vi "Test Helper Loop Restart.vi"(8 "error in (no error)":errorcluster, 11 "Helper Loop Test In":refnum<class "Helper Loop Test.lvclass">) -> (0 "error out":errorcluster, 3 "Helper Loop Test Out":refnum<class "Helper Loop Test.lvclass">)   [LabVIEW 2020, in "Helper Loop Test.lvclass"]
uses:
  Helper Loop Test.lvclass
  C:/Program Files (x86)/National Instruments/LabVIEW 2020/vi.lib/Asteme/LUnit/Test Case.lvclass
  Mock Process/Mock Process.lvclass
  C:/Users/anton/Documents/GitHub/Triarc-Framework/source/Framework/Process/Process.lvclass
  <vilib>/Asteme/LUnit/Test Case.lvclass/Test Case.ctl
  <vilib>/Asteme/LUnit/LUnit Assertion Result.lvclass/LUnit Assertion Result.ctl
  Framework/Process/Process.lvclass/Process.ctl
  <vilib>/Asteme/LUnit/Palette/Fail.vi
  <vilib>/Asteme/LUnit/Palette/Pass.vi
  <vilib>/Asteme/LUnit/Set Assertion Type.vi
  Framework/Process/Public/Get Lifecycle State.vi
  Framework/Process/Private/SubVIs/Wait for finish.vi
  Framework/Process/Protected/Messaging/Enqueue Message.vi
  Framework/Process/Private/SubVIs/Set Lifecycle State.vi
  <vilib>/Asteme/LUnit/Add test result.vi
  <vilib>/Asteme/LUnit/LUnit Write Passed.vi
  <vilib>/Asteme/LUnit/LUnit Get Test Case.vi
  <vilib>/Asteme/LUnit/LUnit Write Message.vi
  <vilib>/Asteme/LUnit/LUnit Write Description.vi
  <vilib>/Asteme/LUnit/LUnit Write Assertion Type.vi
  <vilib>/Utility/error.llb/Clear Errors.vi
  <vilib>/Asteme/LUnit/Read Test Case Name.vi
  <vilib>/Asteme/LUnit/Assertion Result/LUnit Get Test Name.vi
  <vilib>/Utility/error.llb/Error Cluster From Error Code.vi
  <vilib>/Asteme/LUnit/LUnit Assertion Result.lvclass
  Framework/Process/Process.lvclass
  <vilib>/Asteme/LUnit/Test Case.lvclass
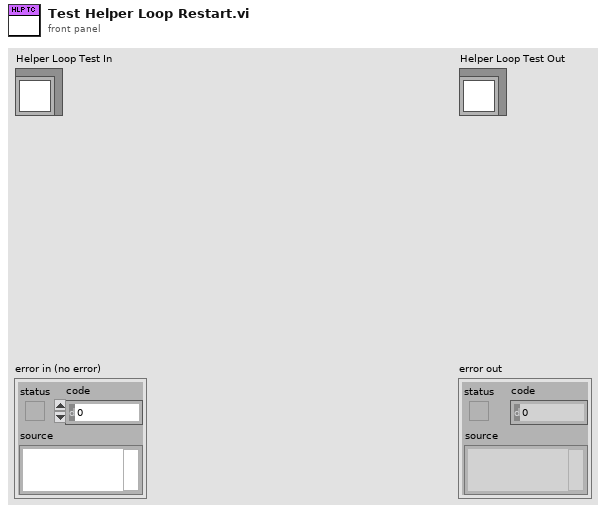
[diagram p1: front panel]
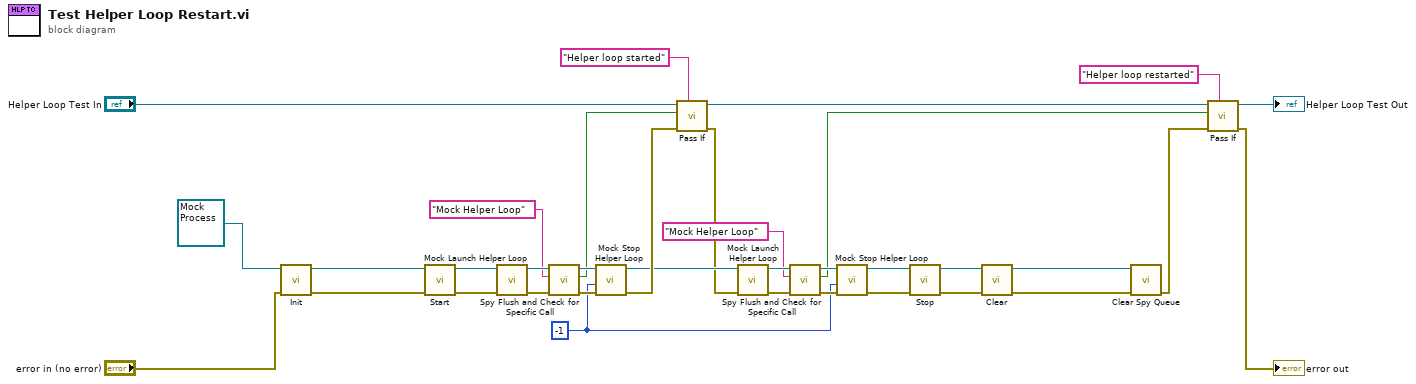
[diagram p0: block diagram]
diagram:
  w1 = -1 ("timeout in ms (-1)")
  n1 = call-dynamic "Init.vi"("error in (no error)"="error in (no error)", "Mock Process In"=refnum<class "Mock Process.lvclass"> refnum) -> ("error out"=w34:errorcluster, "Mock Process Out"=w35:refnum<class "Mock Process.lvclass">)  [unwired: 8 in]
  n2 = call "Start.vi"("error in (no error)"=w34, "Process In"=w35) -> ("error out"=w32:errorcluster, "Process Out"=w33:refnum<class "Mock Process.lvclass">)  [unwired: 8 in]
  n3 = call "Mock Launch Helper Loop.vi"("error in (no error)"=w32, "Mock Process in"=w33) -> ("error out"=w21:errorcluster, "Mock Process out"=w18:refnum<class "Mock Process.lvclass">)  [unwired: 8 in]
  n4 = call "Spy Flush and Check for Specific Call.vi"("error in (no error)"=w21, "Specific Call"="Mock Helper Loop" ("Message"), "Mock Rig Process In"=w18) -> ("error out"=w20:errorcluster, "Occured?"=w15:bool, "Mock Rig Process Out"=w19:refnum<class "Mock Process.lvclass">)  [unwired: 6 in]
  n5 = call "Mock Stop Helper Loop.vi"("error in (no error)"=w20, "timeout in ms (-1)"=w1, "Mock Process in"=w19) -> ("error out"=w13:errorcluster, "Mock Process out"=w8:refnum<class "Mock Process.lvclass">)  [unwired: 6 in, 1 out]
  n6 = call <vilib>:"Pass If.vi"("Description"="Helper loop started", "error in (no error)"=w13, "Pass?"=w15, "Test Case In"="Helper Loop Test In") -> ("error out"=w6:errorcluster, "Test Case Out"=w16:refnum<class "Helper Loop Test.lvclass">)  [unwired: 6 in]
  n7 = call "Mock Launch Helper Loop.vi"("error in (no error)"=w6, "Mock Process in"=w8) -> ("error out"=w9:errorcluster, "Mock Process out"=w12:refnum<class "Mock Process.lvclass">)  [unwired: 8 in]
  n8 = call "Spy Flush and Check for Specific Call.vi"("error in (no error)"=w9, "Specific Call"="Mock Helper Loop" ("Message"), "Mock Rig Process In"=w12) -> ("error out"=w10:errorcluster, "Occured?"=w2:bool, "Mock Rig Process Out"=w11:refnum<class "Mock Process.lvclass">)  [unwired: 6 in]
  n9 = call "Mock Stop Helper Loop.vi"("error in (no error)"=w10, "timeout in ms (-1)"=w1, "Mock Process in"=w11) -> ("error out"=w5:errorcluster, "Mock Process out"=w7:refnum<class "Mock Process.lvclass">)  [unwired: 6 in, 1 out]
  n10 = call "Stop.vi"("error in (no error)"=w5, "Process In"=w7) -> ("error out"=w30:errorcluster, "Process Out"=w31:refnum<class "Mock Process.lvclass">)  [unwired: 7 in, 1 out]
  n11 = call-dynamic "Clear.vi"("error in (no error)"=w30, "Mock Process In"=w31) -> ("error out"=w28:errorcluster, "Mock Process Out"=w29:refnum<class "Mock Process.lvclass">)  [unwired: 8 in]
  n12 = call-dynamic "Clear Spy Queue.vi"("error in (no error)"=w28, "Mock Process In"=w29) -> ("error out"=w24:errorcluster)  [unwired: 8 in, 1 out]
  n13 = call <vilib>:"Pass If.vi"("Description"="Helper loop restarted", "error in (no error)"=w24, "Pass?"=w2, "Test Case In"=w16) -> ("error out"=→"error out":errorcluster, "Test Case Out"=→"Helper Loop Test Out":refnum<class "Helper Loop Test.lvclass">)  [unwired: 6 in]
